vi "Read Data Rate.vi"(8 "error in":errorcluster, 11 "objects":T1) -> (0 "error out":errorcluster, 2 "Rate":dbl)   [LabVIEW 2014, in "DAQmx Module Editor Node.lvclass"]
uses:
  DAQmx Module Editor Node.lvclass
  <vilib>/NI/DCAF/Tag Editor Core/Table API/Table Manager/object ref.ctl
  <vilib>/NI/DCAF/Tag Editor Core/Configuration Editor/Classes/Engine Parent/Engine Parent Editor Node.lvclass
  <vilib>/NI/DCAF/Tag Editor Core/Configuration Editor/Classes/Module editor node/module editor node.lvclass
  module/configuration/DAQmx Module Configuration.lvclass/DAQmx Module Configuration.ctl
  module/configuration/DAQmx Module Configuration.lvclass
  <vilib>/NI/DCAF/Tag Editor Core/Table API/Table Manager/Table Manager.lvclass
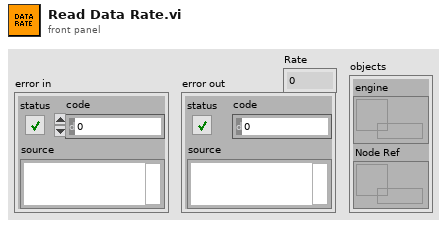
[diagram p1: front panel]
types:
  T1 = typedef "Table Manager.lvlib/Table Manager.lvclass/object ref.ctl" = cluster{"engine":refnum<data-value>, "Node Ref":refnum<data-value>}
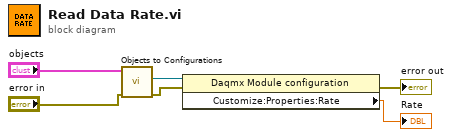
[diagram p0: block diagram]
diagram:
  n1 = call "Objects to Configurations.vi"("error in (no error)"="error in", "Objects in"="objects") -> ("error out"=w3:errorcluster, "tag bus configurable plugin module configuration"=w6:refnum<class "DAQmx Module Configuration.lvclass">)  [unwired: 7 in, 1 out]
  n2 = property class="Daqmx Module configuration"(reference=w6, error in=w3) -> (error out=→"error out":errorcluster, "Customize:Properties:Rate"=→"Rate":dbl)  [unwired: 1 out]
